vi "ConstructConfigFilePath.vi"(8 "error in (no error)":errorcluster, 11 "Reference to calling VI":refnum<vi>) -> (0 "error out":errorcluster, 2 "appended path":path)   [LabVIEW 2013]
uses:
  Special Folder Enum.ctl
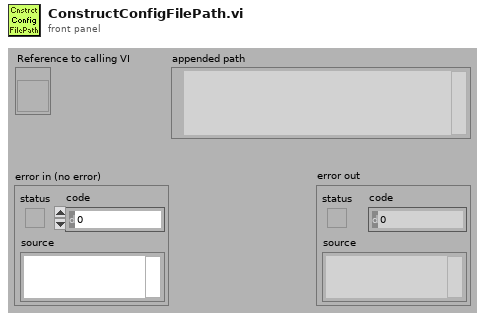
[diagram p1: front panel]
types:
  T1 = typedef "Special Folder Enum.ctl" = enum32{"Desktop", "Err<Internet>", "Programs", "Err<Controls>", "Err<Printers>", "Personal (MyDocuments)", "Favorites", "Startup", "Recent", "SendTo", "Err<RecycleBin>", "StartMenu", "Err<MyDocuments>", "MyMusic", "MyVideo", "Err<0x000F>", "DesktopDirectory", "Err<Drives>", "Err<Network>", "NetHood", "Fonts", "Templates", "CommonStartMenu", "CommonPrograms", "CommonStartup", "CommonDesktopDirectory", "AppData", "PrintHood", "LocalAppData", "Err<AltStartup>", "Err<CommonAltStartup>", "CommonFavorites", "InternetCache", "Cookies", "History", "CommonAppData", "Windows", "System", "ProgramFiles", "MyPictures", "Profile", "System32", "Err<0x002A>", "ProgramFilesCommon", "Err<0x002C>", "CommonTemplates", "CommonDocuments", "CommonAdminTools", "AdminTools"}
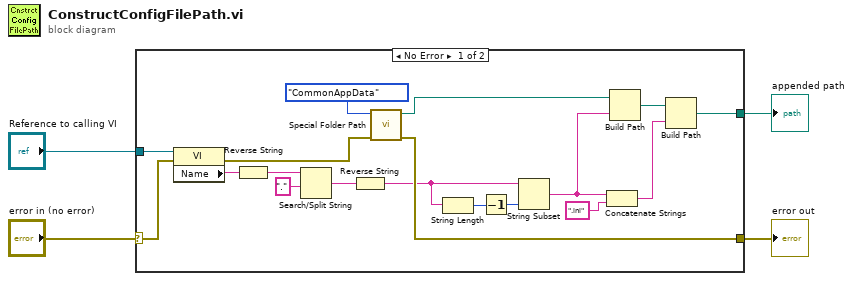
[diagram p0: block diagram]
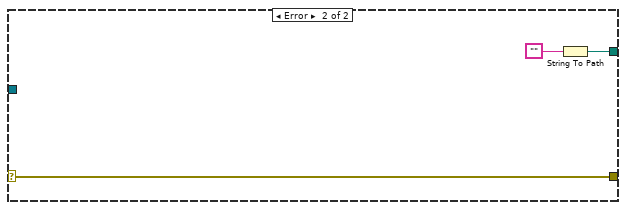
[diagram p2: hidden frame]
diagram:
  n1 = case shown="No Error" "error in (no error)" {
    selector: "error in (no error)" -> [w12 w25]
    tunnel: [w22 w24] -> w4
    tunnel: "Reference to calling VI" -> [w17 _]
    tunnel: [w10 w25] -> w1
    frame No Error {
      n2 = property class="VI"(reference=w17, error in=w12) -> (error out=w11:errorcluster, "Name"=w18:string)  [unwired: 1 out]
      n3 = Reverse String(1:w18) -> (0:w14:string)
      n4 = Search/Split String(string=w14, search string/char (-)=".") -> (match + rest of string=w13:string)  [unwired: 1 in, 2 out]
      n5 = Reverse String(1:w13) -> (0:w7:string)
      n6 = call "Special Folder Path.vi"("error in (no error)"=w11, "Special Folder"=Special_Folder_Enum."CommonAppData") -> ("error out"=w10:errorcluster, "Path"=w9:path)  [unwired: 8 in]
      n7 = String Length(string=w7) -> (length=w6:i32)
      n8 = Decrement(x=w6) -> (x-1=w5:i32)
      n9 = String Subset(string=w7, length (rest)=w5) -> (substring=w8:string)  [unwired: 1 in]
      n10 = Concatenate Strings(w8, ".ini" ("name or relative path")) -> (w21:string)
      n11 = Build Path(base path=w9, name or relative path=w8) -> (appended path=w16:path)
      n12 = Build Path(base path=w16, name or relative path=w21) -> (appended path=w22:path)
    }
    frame Error {
      n13 = String To Path(string="") -> (path=w24:path)
    }
  }
  "appended path" <- w4
  "error out" <- w1
